vi "Get Thread Interfaces Pool.vi"(11 "Plugin in":refnum<class "Plugin.lvclass">) -> (2 "Plugin Interfaces Pool":refnum<class "Plugin Interface Pool.lvclass">, 3 "Plugin out":refnum<class "Plugin.lvclass">)   [LabVIEW 2017, in "DSF Core.lvlib" / "Plugin.lvclass"]
uses:
  Plugin.lvclass
  Thread Pool/Plugin Interface Pool.lvclass
  Plugin.lvclass/Plugin.ctl
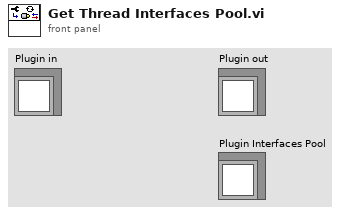
[diagram p1: front panel]
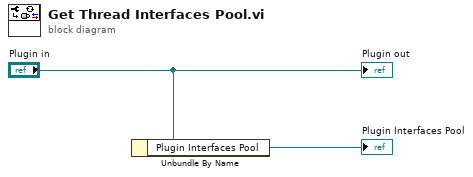
[diagram p0: block diagram]
diagram:
  n1 = Unbundle By Name("Plugin in") -> ("Plugin Interfaces Pool"=→"Plugin Interfaces Pool":refnum<class "Plugin Interface Pool.lvclass">)
  "Plugin out" <- "Plugin in"
